vi "AO Write.vi"(8 "error in (no error)":errorcluster, 10 "Params":variant, 11 "NI Analog Output in":refnum<class "NI Analog Output.lvclass">) -> (0 "error out":errorcluster, 3 "NI Analog Output out":refnum<class "NI Analog Output.lvclass">)   [LabVIEW 2020, in "NI DAQmx.lvlib" / "NI Analog Output.lvclass"]
uses:
  NI Analog Output.lvclass
  D:/WSGitHub/RTFWK/Realization/NI DAQmx Base/NI DAQmx Base.lvclass
  TypeDefs/Output Config.ctl
  <vilib>/DAQmx/write.llb/DAQmx Write (Analog DBL 1Chan 1Samp).vi
  <vilib>/DAQmx/write.llb/DAQmx Write (Analog 1D DBL 1Chan NSamp).vi
  <vilib>/DAQmx/write.llb/DAQmx Write (Analog 2D DBL NChan NSamp).vi
  <vilib>/DAQmx/write.llb/DAQmx Write (Analog 1D DBL NChan 1Samp).vi
  <vilib>/DAQmx/miscellaneous.llb/DAQmx Fill In Error Info.vi
  <resource>/objmgr/daqmx.rc
  <vilib>/Utility/Data Type/NI_Data Type.lvlib
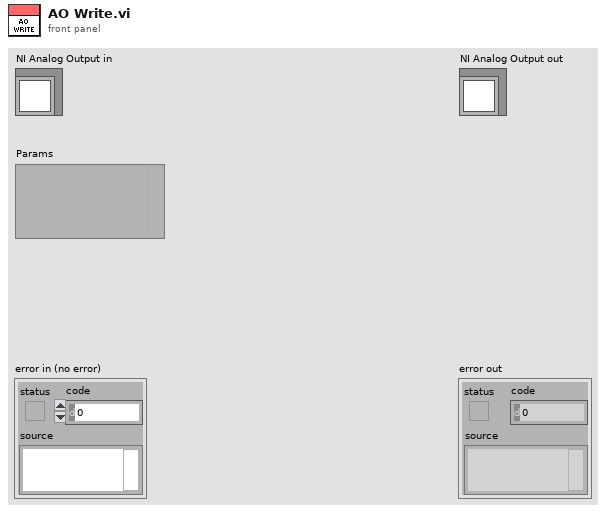
[diagram p1: front panel]
types:
  T1 = typedef "Output Config.ctl" = cluster{"data":variant, "auto start":bool, "regeneration":bool}
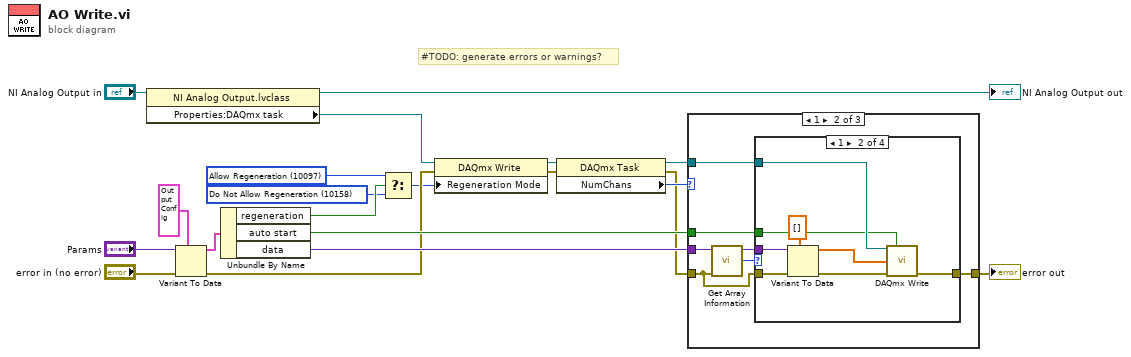
[diagram p0: block diagram]
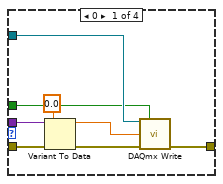
[diagram p3: hidden frame]
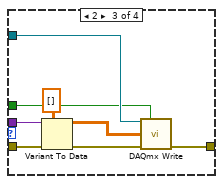
[diagram p4: hidden frame]
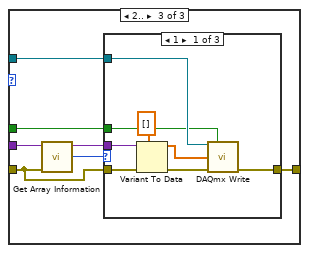
[diagram p6: hidden frame]
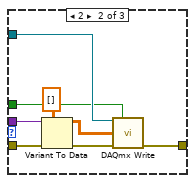
[diagram p7: hidden frame]
diagram:
  w1 = 10158 items=["Allow Regeneration"=10097, "Do Not Allow Regeneration"=10158] ("RegenMode")
  w3 = 10097 items=["Allow Regeneration"=10097, "Do Not Allow Regeneration"=10158] ("RegenMode")
  # "#TODO: generate errors or warnings?"
  n1 = property class="NI Analog Output.lvclass"(reference="NI Analog Output in") -> (reference out=→"NI Analog Output out":refnum<class "NI Analog Output.lvclass">, "Properties:DAQmx task"=w8:refnum<k21>)  [unwired: 1 in, 1 out]
  n2 = Variant To Data(error in="error in (no error)", type=T1 {"data"=variant, "auto start"=FALSE, "regeneration"=FALSE}, Variant="Params") -> (data=w5:T1, error out=w7:errorcluster)
  n3 = Unbundle By Name(w5) -> ("regeneration"=w2:bool, "auto start"=w11:bool, "data"=w12:variant)
  n4 = Select(t=w3, s=w2, f=w1) -> (s? t:f=w4:i32)
  n5 = property class="DAQmx Write"(reference=w8, error in=w7, "Regeneration Mode"=w4) -> (reference out=w10:refnum<k21>, error out=w9:errorcluster)
  n6 = property class="DAQmx Task"(reference=w10, error in=w9) -> (reference out=w14:refnum<k21>, error out=w6:errorcluster, "NumChans"=w13:u32)
  n7 = case shown="1" w13 {
    tunnel: [w21 w27 w58] -> w15
    tunnel: w6 -> [w21 w22 w53]
    tunnel: w12 -> [_ w24 w55]
    tunnel: w14 -> [_ w26 w57]
    tunnel: w11 -> [_ w23 w54]
    frame 0, Default {
      # "no channels in task"
    }
    frame 1 {
      n8 = call <vilib>:"Get Array Information.vi"("error in (no error)"=w22, "variant"=w24) -> ("number of dimensions"=w25:i32)  [unwired: 6 in, 3 out]
      n9 = case shown="1" w25 {
        tunnel: [w32 w43 w51 w52] -> w27
        tunnel: w26 -> [w31 w41 w49 _]
        tunnel: w24 -> [w30 w38 w46 _]
        tunnel: w23 -> [w29 w37 w45 _]
        tunnel: w22 -> [w28 w36 w44 w52]
        frame 0 {
          n10 = Variant To Data(error in=w28, type=0.0 ("Numeric"), Variant=w30) -> (data=w34:dbl, error out=w35:errorcluster)
          n11 = call-poly <vilib>:"DAQmx Write.vi"("task/channels in"=w31, "auto start"=w29, "data"=w34, "error in"=w35) -> ("error out"=w32:errorcluster)  [unwired: 9 in, 2 out]
        }
        frame 1 {
          n12 = Variant To Data(error in=w36, type=dbl[] [] ("Numeric"), Variant=w38) -> (data=w40:dbl[], error out=w42:errorcluster)
          n13 = call-poly <vilib>:"DAQmx Write.vi"("task/channels in"=w41, "auto start"=w37, "data"=w40, "error in"=w42) -> ("error out"=w43:errorcluster)  [unwired: 9 in, 2 out]
        }
        frame 2 {
          n14 = Variant To Data(error in=w44, type=dbl[][] [] ("Numeric"), Variant=w46) -> (data=w48:dbl[][], error out=w50:errorcluster)
          n15 = call-poly <vilib>:"DAQmx Write.vi"("task/channels in"=w49, "auto start"=w45, "data"=w48, "error in"=w50) -> ("error out"=w51:errorcluster)  [unwired: 9 in, 2 out]
        }
        frame Default {
          # "invalid data type"
        }
      }
    }
    frame 2.. {
      n16 = call <vilib>:"Get Array Information.vi"("error in (no error)"=w53, "variant"=w55) -> ("number of dimensions"=w56:i32)  [unwired: 6 in, 3 out]
      n17 = case shown="1" w56 {
        tunnel: [w66 w74 w75] -> w58
        tunnel: w57 -> [w64 w72 _]
        tunnel: w55 -> [w60 w68 _]
        tunnel: w54 -> [w61 w69 _]
        tunnel: w53 -> [w59 w67 w75]
        frame 1 {
          n18 = Variant To Data(error in=w59, type=dbl[] [] ("Numeric"), Variant=w60) -> (data=w63:dbl[], error out=w65:errorcluster)
          n19 = call-poly <vilib>:"DAQmx Write.vi"("task/channels in"=w64, "auto start"=w61, "data"=w63, "error in"=w65) -> ("error out"=w66:errorcluster)  [unwired: 9 in, 2 out]
        }
        frame 2 {
          n20 = Variant To Data(error in=w67, type=dbl[][] [] ("Numeric"), Variant=w68) -> (data=w71:dbl[][], error out=w73:errorcluster)
          n21 = call-poly <vilib>:"DAQmx Write.vi"("task/channels in"=w72, "auto start"=w69, "data"=w71, "error in"=w73) -> ("error out"=w74:errorcluster)  [unwired: 9 in, 2 out]
        }
        frame Default {
        }
      }
    }
  }
  "error out" <- w15
